vi "Add ColumnHead Item by Text Width TextAlign and ImageIndex.vi"(6 "imageIndex":i32, 7 "textAlign":i32(ring) items=["Left", "Right", "Center"], 8 "error in (no error)":errorcluster caption="错误输入（无错误）", 9 "width":i32, 10 "text":string, 11 "ListViewClass 输入":refnum<class "ListViewClass.lvclass"> caption="DNL_LabVIEW Object in") -> (0 "error out":errorcluster caption="错误输出", 3 "ListViewClass 输出":refnum<class "ListViewClass.lvclass"> caption="DNL_LabVIEW Object out")   [LabVIEW 2012, in "ListViewClass.lvclass"]
uses:
  ListViewClass.lvclass
  ListViewClass.lvclass/ListViewClass.ctl
  System.Windows.Forms
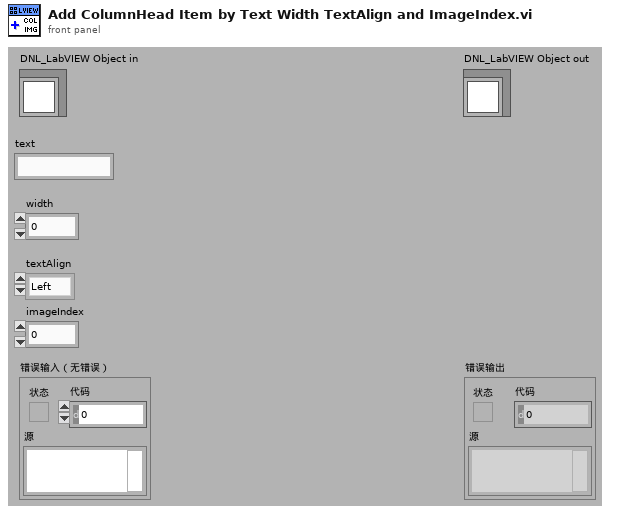
[diagram p1: front panel]
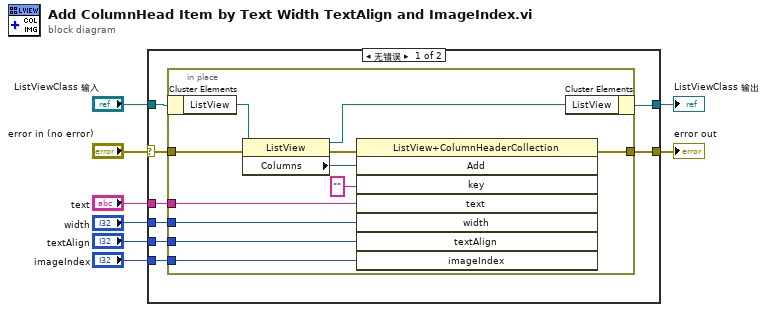
[diagram p0: block diagram]
diagram:
  n1 = case shown="无错误" "error in (no error)" {
    selector: "error in (no error)" -> [w10 w29]
    tunnel: [w9 w29] -> w7
    tunnel: [w15 w28] -> w5
    tunnel: "ListViewClass 输入" -> [w16 w28]
    tunnel: "text" -> [w14 _]
    tunnel: "width" -> [w13 _]
    tunnel: "textAlign" -> [w12 _]
    tunnel: "imageIndex" -> [w11 _]
    frame No Error {
      n2 = in-place {
        in-place-border: w14 -> [w25]
        in-place-border: w13 -> [w24]
        in-place-border: w12 -> [w23]
        in-place-border: w11 -> [w22]
        in-place-border: w10 -> [w20]
        in-place-border: [w17] -> w9
        n3 = in-place-cluster #1(w16) -> ("ListView"=w27:refnum<k24>)
        n4 = property class="ListView"(reference=w27, error in=w20) -> (reference out=w19:refnum<k24>, error out=w18:errorcluster, "Columns"=w21:refnum<k24>)
        n5 = invoke class="ListView+ColumnHeaderCollection" method="Add"(reference=w21, error in=w18, "key"="", "text"=w25, "width"=w24, "textAlign"=w23, "imageIndex"=w22) -> (error out=w17:errorcluster)  [unwired: 1 in, 7 out]
        n6 = in-place-cluster #1("ListView"=w19) -> (w15:refnum<class "ListViewClass.lvclass">)
      }
    }
    frame Error {
    }
  }
  "error out" <- w7
  "ListViewClass 输出" <- w5
